vi "PH_Strings.select string from array.vi"(2 "String Array in":string[](array[string]), 4 "Caption.Text":string, 5 "error in (no error)":errorcluster) -> (16 "string out":string, 17 "index":i32, 19 "error out":errorcluster)   [LabVIEW 2014, in "PH_Common.lvlib"]
doc: "This VI is forseen to select a string from an array of strings."
uses:
  PH_Common.lvlib
panel:
  in  "Cancel":bool
  in  "OK Button":bool
  in  "Choice":u16(ring) caption="Black Boxes" items=["COS_Test_BB", "Exp_1_BB", "Exp_2_BB", "Exp_3_BB", "Exp_4_BB", "MAS_Test_BB", "NS_Switch_PA_BB", "Test_BB16_BB", "Test_MA_BB", "Z6_ST_100TW_BL_TB_2_CH_BB", "Z6_ST_Comp_Input_CH_BB", "Z6_ST_Comp_Output_CH_BB", "Z6_ST_Comp_Output_Screen_BB", "Z6_TA_100TW_BL_TB_3_CH_BB"]
  # "PCS"
  # "3.40"
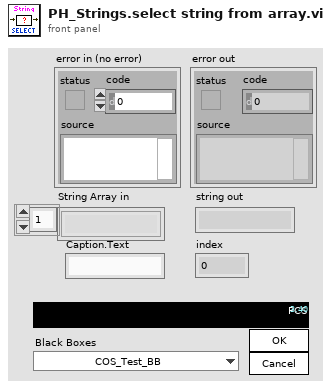
[diagram p1: front panel]
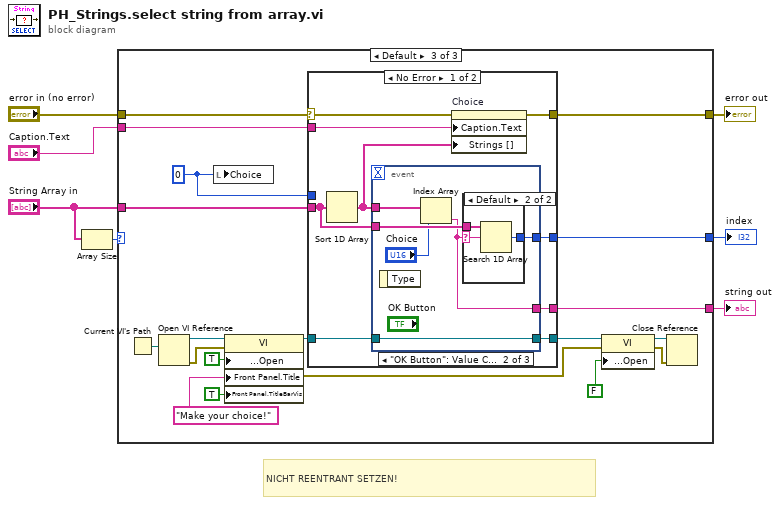
[diagram p0: block diagram]
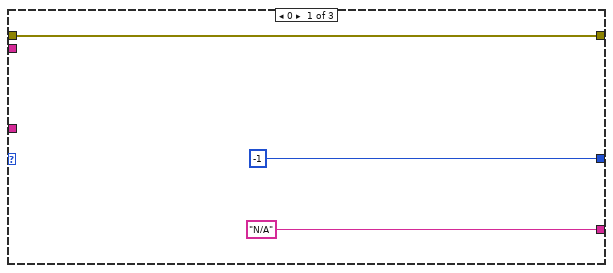
[diagram p2: hidden frame]
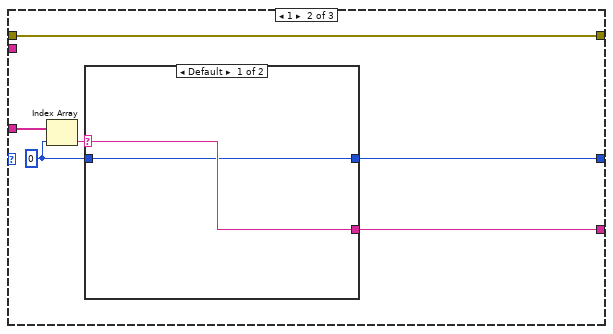
[diagram p3: hidden frame]
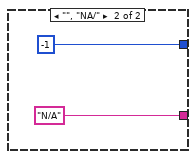
[diagram p4: hidden frame]
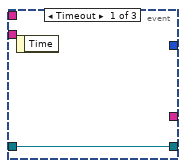
[diagram p5: hidden frame]
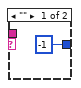
[diagram p6: hidden frame]
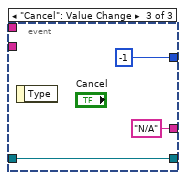
[diagram p7: hidden frame]
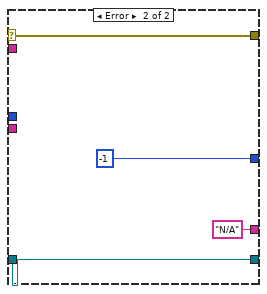
[diagram p8: hidden frame]
diagram:
  # "NICHT REENTRANT SETZEN!"
  n1 = Array Size(array="String Array in") -> (size(s)=w1:i32)
  n2 = case shown="Default" w1 {
    tunnel: ["N/A" ("String") w14 w39] -> w7
    tunnel: "String Array in" -> [_ w13 w38]
    tunnel: [w10 w16 w37] -> w6
    tunnel: "error in (no error)" -> [w10 w16 w26]
    tunnel: [-1 ("Items") w15 w25] -> w4
    tunnel: "Caption.Text" -> [_ _ w23]
    frame 0 {
    }
    frame 1 {
      w11 = 0 ("index")
      n3 = Index Array(array=w13, index=w11) -> (element=w12:string)
      n4 = case shown="Default" w12 {
        selector: w12 -> [w18 _]
        tunnel: [w17 -1 ("Items")] -> w15
        tunnel: [w18 "N/A" ("String")] -> w14
        tunnel: w11 -> [w17 _]
        frame Default {
        }
        frame "", "NA/" {
        }
      }
    }
    frame Default {
      w24 = 0
      n5 = Current VI's Path() -> (path=w36:path)
      n6 = Open VI Reference(vi path=w36) -> (vi reference=w35:refnum<vi>, error out=w29:errorcluster)  [unwired: 5 in]
      n7 = local write "Choice"(w24) -> ()
      n8 = property class="VI"(reference=w35, error in=w29, "Front Panel Window:Open"=TRUE, "Front Panel.Title"="Make your choice!" ("Front Panel Window:Title"), "Front Panel.TitleBarVis"=TRUE ("Front Panel Window:Title Bar Visible")) -> (reference out=w33:refnum<vi>, error out=w28:errorcluster)
      n9 = case shown="No Error" w26 {
        selector: w26 -> [w44 w66]
        tunnel: [w48 "N/A" ("String")] -> w39
        tunnel: w38 -> [w42 _]
        tunnel: [w47 w66] -> w37
        tunnel: w33 -> [w46 w65]
        tunnel: [w45 w65] -> w31
        tunnel: [w43 -1 ("Items")] -> w25
        tunnel: w24 -> [_ _]
        tunnel: w23 -> [w40 _]
        frame No Error {
          n10 = Sort 1D Array(array=w42) -> (sorted array=w41:string[])
          n11 = event shown="[1] \"OK Button\": Value Change" {
            selector: _ -> [_ _ _]
            dyn-events: _ -> [_ _ _]
            timeout: _ -> [_ _ _]
            tunnel: w41 -> [_ w55 _]
            tunnel: [_ w50 "N/A" ("String")] -> w48
            tunnel: [w49 w54 w62] -> w45
            tunnel: w46 -> [w49 w54 w62]
            tunnel: [_ w51 -1 ("Items")] -> w43
            tunnel: w42 -> [_ w53 _]
            event Timeout {
              n12 = event-data() -> ()  [unwired: 1 in, 1 out]
            }
            event "OK Button": Value Change {
              n13 = event-data() -> ()  [unwired: 1 in, 1 out]
              n14 = Index Array(array=w55, index="Choice") -> (element=w50:string)
              n15 = case shown="Default" w50 {
                selector: w50 -> [_ w57]
                tunnel: w53 -> [_ w59]
                tunnel: [-1 ("index of element") w58] -> w51
                frame "" {
                }
                frame Default {
                  n16 = Search 1D Array(1D array=w59, element=w57) -> (index of element=w58:i32)  [unwired: 1 in]
                }
              }
            }
            event "Cancel": Value Change {
              n17 = event-data() -> ()  [unwired: 1 in, 1 out]
            }
          }
          n18 = property on="Choice" class="Ring (strict)"(error in=w44, "Caption.Text"=w40, "Strings []"=w41) -> (error out=w47:errorcluster)  [unwired: 1 in, 1 out]
        }
        frame Error {
        }
      }
      n19 = property class="VI"(reference=w31, error in=w28, "Front Panel Window:Open"=FALSE) -> (reference out=w30:refnum<vi>, error out=w27:errorcluster)
      n20 = Close Reference(reference=w30, error in (no error)=w27) -> ()  [unwired: 1 out]
    }
  }
  "error out" <- w6
  "string out" <- w7
  "index" <- w4
